vi "PH_ImageCoG_Plotter.panel.vi"(0 "object ref":refnum<vi>, 5 "error in (no error)":errorcluster) -> (19 "error out":errorcluster)   [LabVIEW 2014, in "PH_ImageCoG_Plotter.lvlib"]
doc: "The voltage measured by a device on high potential is represented by a frequency given out by a Beckhoff Klemme. This VI transforms it back into a voltage which wich is written to a memory tag. This value is indicated. In case of no connection (not mounted or bad tag value) or internal problems \"99999\" apears.\n\n\"Exit\" closes the GUI while \"Delete Instance\" additionally destroys the Instance.\n\n\n\nLicense Agreement for this software:\n\nCopyright (C)\nGesellschaft für Schwerionenforschung, GSI\nPlanckstr. 1\n64291 Darmstadt\nGermany\n\nContact: D.Beck@gsi.de \n\nThis program is free software; you can redistribute it and/or modify it under the terms of the GNU General Public License as published by the Free Software Foundation; either version 2 of the license, or (at your option) any later version.\n\nThis program is distributed in the hope that it will be useful, but WITHOUT ANYW ARRANTY; without even the implied warranty of MERCHANTABILITY or FITNESS FOR A PARTICULAR PURPOSE. See the GNU General License for more details (http://www.gnu.org).\n\nGesellschaft für Schwerionenforschung, GSI\nPlanckstr. 1, 64291 Darmstadt, Germany\nFor all questions and ideas contact: M.Richter@gsi.de, H.Brand@gsi.de or D.Beck@gsi.de.\nLast update: 18-DEC-2002"
uses:
  PH_ImageCoG_Plotter.lvlib
  PH_ImageCalibrator/PH_ImageCalibrator.Calibration Data.ctl
  PH_Basics/PH_Img_BaseClass/PH_Img_BaseClass.Palette.ctl
  PH_Basics/PH_Img_BaseClass/PH_Img_BaseClass.GUI Refs.ctl
  CS_Core/CSObj/CSObj.lvlib
  CS_Core/CSSystem/CSSystemLib/CSSystemLib.lvlib
  PH_Basics/PH_Common/PH_Common.lvlib
  PH_Basics/PH_Img_BaseClass/PH_Img_BaseClass.lvlib
  PH_Basics/PH_Class/PH_Class.lvlib
  PH_ImageCalibrator/PH_ImageCalibrator.lvlib
panel:
  in  "Export Data":bool
  out "BI subtracted":u32(colorbox)=16860 caption="BI subtr."
  out "Calibration status":u32(colorbox)=16860 caption="Calibration"
  out "Timeout":u32(colorbox)=16860
  in  "Tab Control":T1(tab)
  in  "Refresh Cam Search":bool caption="Refresh"
  in  "Available Cams":u16(ring)
  in  "Timeout Set":i32 caption="ms"
  out "Delta - X":dbl caption="Pix"
  out "Delta - Y":dbl caption="Pix"
  in  "Center":bool
  in  "exp - Y":i32 caption="Pix"
  in  "exp - X":i32 caption="Pix"
  in  "Type":bool caption="NF       FF"
  out "CoG - Y":dbl caption="Pix"
  out "CoG - X":dbl caption="Pix"
  in  "calc Beam Analysis":bool caption="On"
  out "CoG Y":cluster{dbl[], dbl[]}[](graph)
  out "CoG X":cluster{dbl[], dbl[]}[](graph)
  out "Delta Y":cluster{dbl[], dbl[]}[](graph)
  out "Delta X":cluster{dbl[], dbl[]}[](graph)
  in  "Palette":T2 items=["Grey", "Binary", "Gradient", "Rainbow", "Temperature"]
  out "GUI Image":T3(plugin-control)
  in  "read calibration data":bool
  out "Calibration data":T4
  in  "Exit":bool
  in  "Delete":bool
  # "PCS"
  # "3.40"
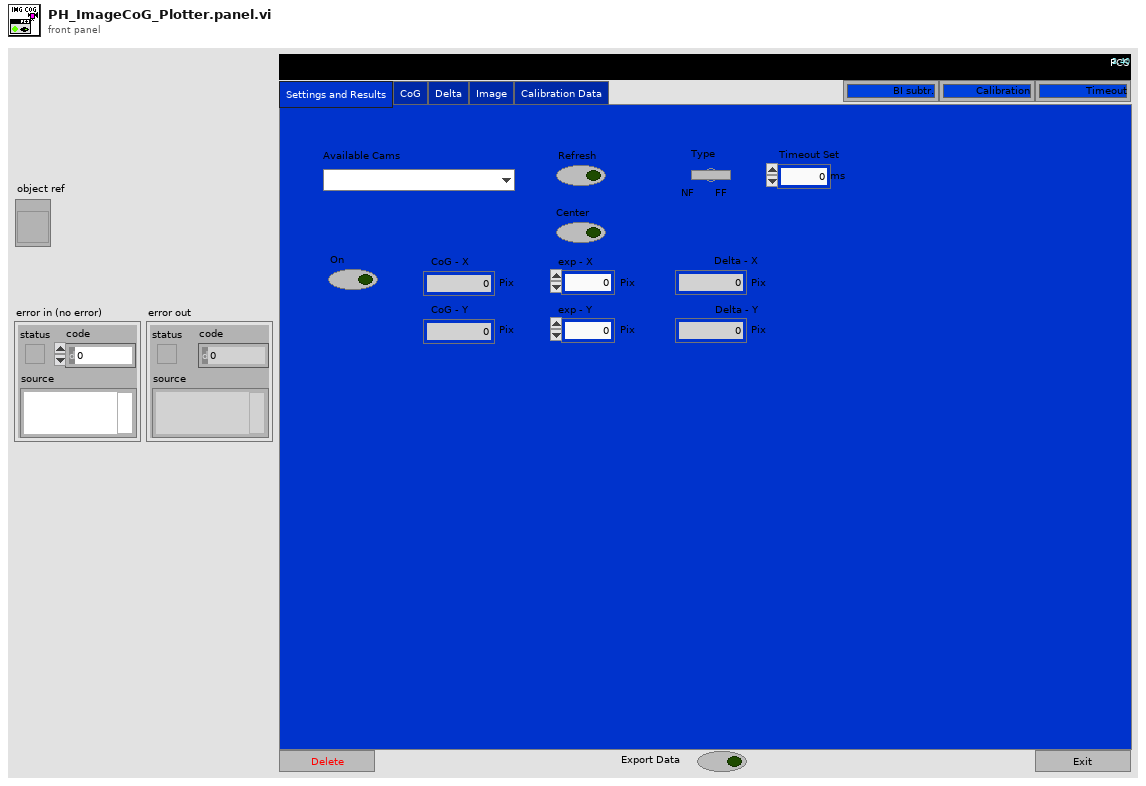
[diagram p1: front panel]
types:
  T1 = enum32{"Settings and Results", "CoG", "Delta", "Image", "Calibration Data"}
  T2 = typedef "PH_Img_BaseClass.lvlib/PH_Img_BaseClass.Palette.ctl" = i32
  T3 = typedef "IMAQ Image.ctl" = refnum<image>
  T4 = typedef "PH_ImageCalibrator.lvlib/PH_ImageCalibrator.Calibration Data.ctl" = cluster{"Date":string, "Time":string, "Cam Settings":cluster{"Cam ID":string, "Gain":dbl, "Brightness":dbl, "Shutter":dbl, "Cam Error":bool, "Mode":i32}, "Background Image":cluster{"Image":dbl[][], "Image Error":bool}, "Linear Calibration":cluster{"Calibration Factor":dbl, "not mm or mrad":bool}, "Energy Calibration":cluster{"Calibration Factor":dbl, "no mJ":bool}}
  T5 = typedef "PH_Img_BaseClass.lvlib/PH_Img_BaseClass.GUI Refs.ctl" = cluster{"Timeout":refnum<vi>, "Image":refnum<vi>, "Palette":refnum<vi>, "Timeout Set":refnum<vi>}
  T6 = typedef "PH_ImageCoG_Plotter.lvlib/PH_ImageCoG_Plotter.i attribute.ctl" = cluster{"GUI Refs":cluster{"Delete":refnum<vi>, "Calibration status":refnum<vi>, "BI subtracted":refnum<vi>, "calc Beam Anal":refnum<vi>, "CoG - x":refnum<vi>, "CoG - y":refnum<vi>, "Type":refnum<vi>, "Center":refnum<vi>, "exp - X":refnum<vi>, "exp - Y":refnum<vi>, "Delta - X":refnum<vi>, "Delta - Y":refnum<vi>, "Available Cams":refnum<vi>, "CoG X":refnum<vi>, "CoG Y":refnum<vi>, "Delta X":refnum<vi>, "Delta Y":refnum<vi>, "Export Data":refnum<vi>, "Calibration data":refnum<vi>}, "Calibration":cluster{"Status":T7, "Calibration data":T4, "Calibration Data File":path}, "Beam Analysis":cluster{"on":bool, "exp - X":i32, "exp - Y":i32, "Type":bool, "Data":cluster{"current time":timestamp, "CoG-x":dbl, "CoG-y":dbl, "Delta-x":dbl, "Delta-y":dbl}[], "Datasets strored":i32, "Dataarray Size":i32}, "Cam instances":string[], "DIM Service Events":T8[], "Images":cluster{"Background":T3, "OP":T3, "GUI":T3}}
  T7 = typedef "PH_StatusHandler.lvlib/PH_StatusHandler.Status.ctl" = i16
  T8 = typedef "BaseProcess.lvlib/BaseProcess.event definition.ctl" = cluster{"CAEEvtDef":T9, "Data Descriptor":T10}
  T9 = typedef "CAEObj.lvlib/CAEObj.event definition.ctl" = cluster{"URL":string, "enable":bool, "ignoreResID":bool}
  T10 = typedef "BaseProcess.lvlib/BaseProcess.descriptor string definition.ctl" = string
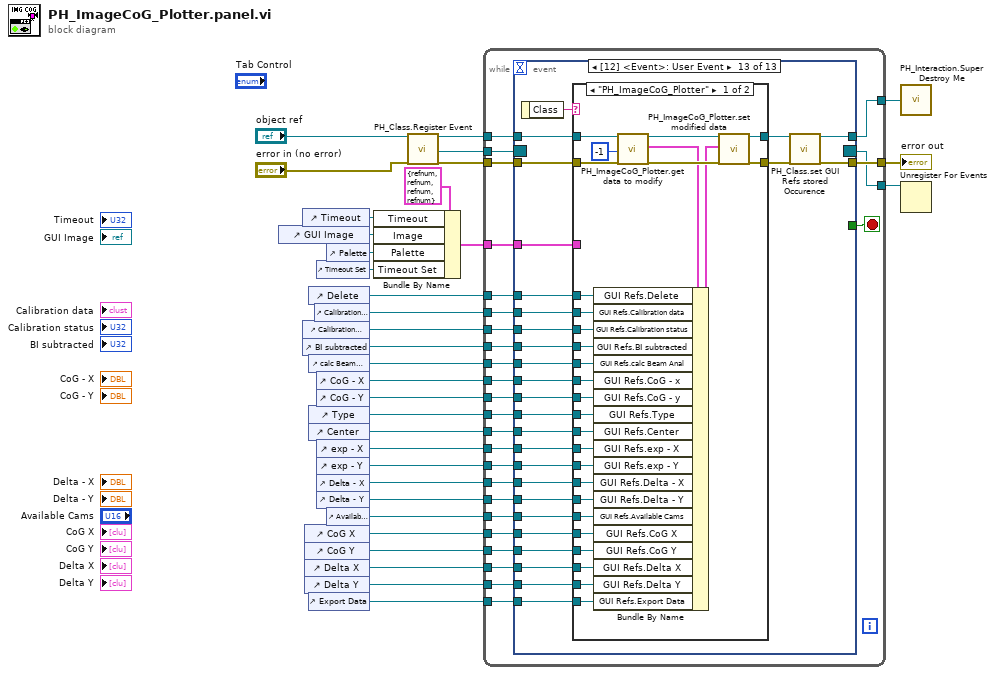
[diagram p0: block diagram]
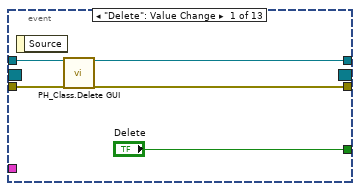
[diagram p2: hidden frame]
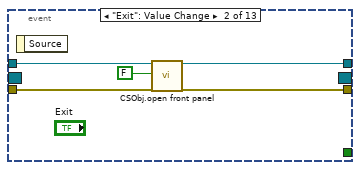
[diagram p3: hidden frame]
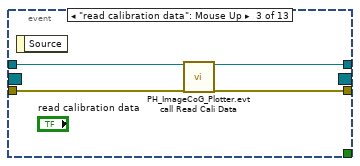
[diagram p4: hidden frame]
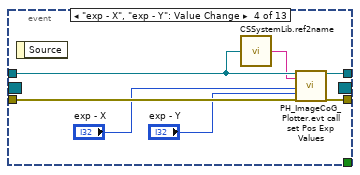
[diagram p5: hidden frame]
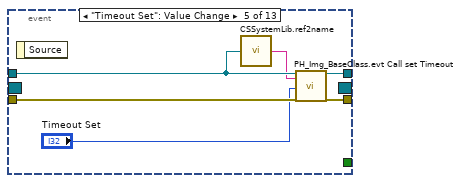
[diagram p6: hidden frame]
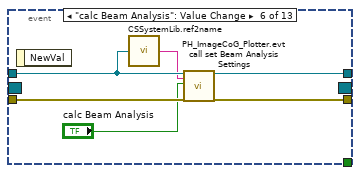
[diagram p7: hidden frame]
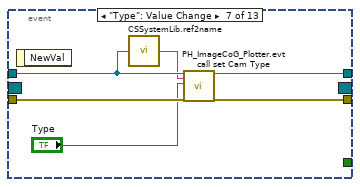
[diagram p8: hidden frame]
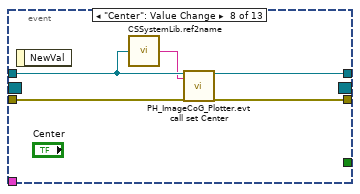
[diagram p9: hidden frame]
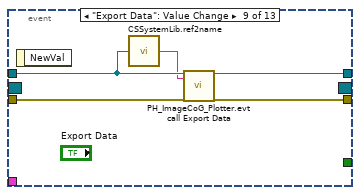
[diagram p10: hidden frame]
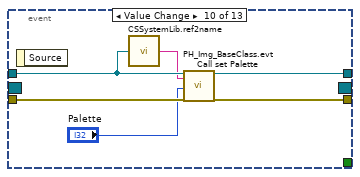
[diagram p11: hidden frame]
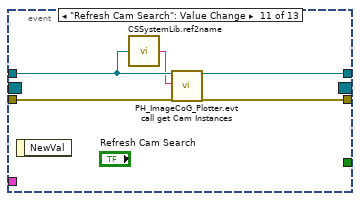
[diagram p12: hidden frame]
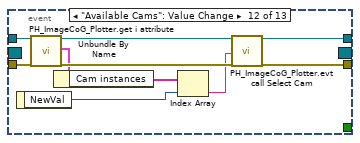
[diagram p13: hidden frame]
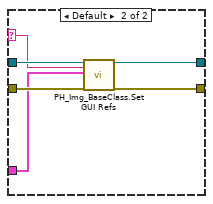
[diagram p14: hidden frame]
diagram:
  n1 = control-ref of="GUI Image"() -> (w29:refnum<vi>)
  n2 = control-ref of="Timeout"() -> (w30:refnum<vi>)
  n3 = control-ref of="Calibration status"() -> (w17:refnum<vi>)
  n4 = control-ref of="BI subtracted"() -> (w16:refnum<vi>)
  n5 = control-ref of="CoG X"() -> (w5:refnum<vi>)
  n6 = control-ref of="CoG Y"() -> (w4:refnum<vi>)
  n7 = control-ref of="Delta X"() -> (w3:refnum<vi>)
  n8 = control-ref of="Delta Y"() -> (w2:refnum<vi>)
  n9 = control-ref of="Delete"() -> (w21:refnum<vi>)
  n10 = control-ref of="calc Beam Analysis"() -> (w15:refnum<vi>)
  n11 = control-ref of="Type"() -> (w12:refnum<vi>)
  n12 = control-ref of="Center"() -> (w11:refnum<vi>)
  n13 = control-ref of="Export Data"() -> (w1:refnum<vi>)
  n14 = control-ref of="Calibration data"() -> (w18:refnum<vi>)
  n15 = control-ref of="Timeout Set"() -> (w27:refnum<vi>)
  n16 = control-ref of="CoG - X"() -> (w14:refnum<vi>)
  n17 = control-ref of="CoG - Y"() -> (w13:refnum<vi>)
  n18 = control-ref of="exp - X"() -> (w10:refnum<vi>)
  n19 = control-ref of="exp - Y"() -> (w9:refnum<vi>)
  n20 = control-ref of="Delta - X"() -> (w8:refnum<vi>)
  n21 = control-ref of="Delta - Y"() -> (w7:refnum<vi>)
  n22 = control-ref of="Palette"() -> (w28:refnum<vi>)
  n23 = control-ref of="Available Cams"() -> (w6:refnum<vi>)
  n24 = Bundle By Name(cluster=T5 {"Timeout"=refnum, "Image"=refnum, "Palette"=refnum, "Timeout Set"=refnum} ("GUI Refs"), "Timeout"=w30, "Image"=w29, "Palette"=w28, "Timeout Set"=w27) -> (w22:T5)
  n25 = call "PH_Class.Register Event.vi"("i ref in"="object ref", "error in (no error)"="error in (no error)") -> ("i ref out"=w26:refnum<vi>, "Event Registration Refnum"=w24:refnum<event-registration>, "error out"=w25:errorcluster)  [unwired: 15 in]
  n26 = while {
    tunnel: w26 -> [w57]
    tunnel: [w56] -> w33
    tunnel: w25 -> [w59]
    tunnel: [w58] -> w32
    tunnel: w24 -> [w55]
    tunnel: [w54] -> w23
    tunnel: w22 -> [w53]
    tunnel: w21 -> [w52]
    tunnel: w18 -> [w51]
    tunnel: w17 -> [w50]
    tunnel: w16 -> [w49]
    tunnel: w15 -> [w48]
    tunnel: w14 -> [w47]
    tunnel: w13 -> [w46]
    tunnel: w12 -> [w45]
    tunnel: w11 -> [w44]
    tunnel: w10 -> [w43]
    tunnel: w9 -> [w42]
    tunnel: w8 -> [w41]
    tunnel: w7 -> [w40]
    tunnel: w6 -> [w39]
    tunnel: w5 -> [w38]
    tunnel: w4 -> [w37]
    tunnel: w3 -> [w36]
    tunnel: w2 -> [w35]
    tunnel: w1 -> [w34]
    stop <- w60 stop-if-true
    n27 = event shown="[12] <Event>: User Event" {
      selector: w55 -> [_ _ _ _ _ _ _ _ _ _ _ _ _]
      dyn-events: [_ _ _ _ _ _ _ _ _ _ _ _ _] -> w54
      timeout: _ -> [_ _ _ _ _ _ _ _ _ _ _ _ _]
      tunnel: ["Delete" _ _ _ _ _ _ _ _ _ _ _ _] -> w60
      tunnel: w57 -> [w64 w69 w74 w78 w84 w90 w96 w101 w106 w112 w118 w128 w157]
      tunnel: w59 -> [w63 w68 w73 w81 w87 w93 w99 w104 w109 w115 w117 w126 w156]
      tunnel: [w61 w67 w71 w79 w85 w91 w97 w102 w107 w113 w120 w129 w149] -> w58
      tunnel: [w62 w66 w72 w80 w86 w92 w98 w103 w108 w114 w119 w130 w150] -> w56
      tunnel: w53 -> [_ _ _ _ _ _ _ _ _ _ _ _ w155]
      tunnel: w52 -> [_ _ _ _ _ _ _ _ _ _ _ _ w153]
      tunnel: w51 -> [_ _ _ _ _ _ _ _ _ _ _ _ w148]
      tunnel: w50 -> [_ _ _ _ _ _ _ _ _ _ _ _ w147]
      tunnel: w49 -> [_ _ _ _ _ _ _ _ _ _ _ _ w146]
      tunnel: w48 -> [_ _ _ _ _ _ _ _ _ _ _ _ w145]
      tunnel: w47 -> [_ _ _ _ _ _ _ _ _ _ _ _ w144]
      tunnel: w46 -> [_ _ _ _ _ _ _ _ _ _ _ _ w143]
      tunnel: w45 -> [_ _ _ _ _ _ _ _ _ _ _ _ w142]
      tunnel: w44 -> [_ _ _ _ _ _ _ _ _ _ _ _ w141]
      tunnel: w43 -> [_ _ _ _ _ _ _ _ _ _ _ _ w140]
      tunnel: w42 -> [_ _ _ _ _ _ _ _ _ _ _ _ w139]
      tunnel: w41 -> [_ _ _ _ _ _ _ _ _ _ _ _ w138]
      tunnel: w40 -> [_ _ _ _ _ _ _ _ _ _ _ _ w137]
      tunnel: w39 -> [_ _ _ _ _ _ _ _ _ _ _ _ w136]
      tunnel: w38 -> [_ _ _ _ _ _ _ _ _ _ _ _ w135]
      tunnel: w37 -> [_ _ _ _ _ _ _ _ _ _ _ _ w134]
      tunnel: w36 -> [_ _ _ _ _ _ _ _ _ _ _ _ w133]
      tunnel: w35 -> [_ _ _ _ _ _ _ _ _ _ _ _ w132]
      tunnel: w34 -> [_ _ _ _ _ _ _ _ _ _ _ _ w131]
      event "Delete": Value Change {
        n28 = event-data() -> ()  [unwired: 1 in, 1 out]
        n29 = call "PH_Class.Delete GUI.vi"("VI in"=w64, "error in (no error)"=w63) -> ("VI out"=w62:refnum<vi>, "error out"=w61:errorcluster)  [unwired: 16 in]
      }
      event "Exit": Value Change {
        n30 = event-data() -> ()  [unwired: 1 in, 1 out]
        n31 = call "CSObj.open front panel.vi"("i ref in"=w69, "frontPanelOpen"=FALSE ("front panel open"), "error in (no error)"=w68) -> ("i ref out"=w66:refnum<vi>, "error out"=w67:errorcluster)  [unwired: 15 in]
      }
      event "read calibration data": Mouse Up {
        n32 = event-data() -> ()  [unwired: 1 in, 1 out]
        n33 = call "PH_ImageCoG_Plotter.evt call Read Cali Data.vi"("i ref in"=w74, "error in"=w73) -> ("i ref out"=w72:refnum<vi>, "error out"=w71:errorcluster)  [unwired: 16 in]
      }
      event "exp - X", "exp - Y": Value Change {
        n34 = event-data() -> ()  [unwired: 1 in, 1 out]
        n35 = call "CSSystemLib.ref2name.vi"("obj refnum"=w78) -> ("name"=w77:string)
        n36 = call "PH_ImageCoG_Plotter.evt call set Pos Exp Values.vi"("i ref in"=w78, "Instance"=w77, "expected value  x [Pix]"="exp - X", "expected value y [Pix]"="exp - Y", "error in (no error)"=w81) -> ("i ref out"=w80:refnum<vi>, "error out"=w79:errorcluster)  [unwired: 13 in]
      }
      event "Timeout Set": Value Change {
        n37 = event-data() -> ()  [unwired: 1 in, 1 out]
        n38 = call "CSSystemLib.ref2name.vi"("obj refnum"=w84) -> ("name"=w83:string)
        n39 = call "PH_Img_BaseClass.evt Call set Timeout.vi"("i ref in"=w84, "Instance"=w83, "Timeout [ms]"="Timeout Set", "error in (no error)"=w87) -> ("i ref out"=w86:refnum<vi>, "error out"=w85:errorcluster)  [unwired: 14 in]
      }
      event "calc Beam Analysis": Value Change {
        n40 = event-data() -> ()  [unwired: 1 in, 1 out]
        n41 = call "CSSystemLib.ref2name.vi"("obj refnum"=w90) -> ("name"=w89:string)
        n42 = call "PH_ImageCoG_Plotter.evt call set Beam Analysis Settings.vi"("i ref in"=w90, "Instance"=w89, "Calculate"="calc Beam Analysis", "error in (no error)"=w93) -> ("i ref out"=w92:refnum<vi>, "error out"=w91:errorcluster)  [unwired: 14 in]
      }
      event "Type": Value Change {
        n43 = event-data() -> ()  [unwired: 1 in, 1 out]
        n44 = call "CSSystemLib.ref2name.vi"("obj refnum"=w96) -> ("name"=w95:string)
        n45 = call "PH_ImageCoG_Plotter.evt call set Cam Type.vi"("i ref in"=w96, "Instance"=w95, "Cam Type"="Type", "error in (no error)"=w99) -> ("i ref out"=w98:refnum<vi>, "error out"=w97:errorcluster)  [unwired: 14 in]
      }
      event "Center": Value Change {
        n46 = event-data() -> ()  [unwired: 1 in, 1 out]
        n47 = call "CSSystemLib.ref2name.vi"("obj refnum"=w101) -> ("name"=w100:string)
        n48 = call "PH_ImageCoG_Plotter.evt call set Center.vi"("i ref in"=w101, "Instance"=w100, "error in (no error)"=w104) -> ("i ref out"=w103:refnum<vi>, "error out"=w102:errorcluster)  [unwired: 15 in]
      }
      event "Export Data": Value Change {
        n49 = event-data() -> ()  [unwired: 1 in, 1 out]
        n50 = call "CSSystemLib.ref2name.vi"("obj refnum"=w106) -> ("name"=w105:string)
        n51 = call "PH_ImageCoG_Plotter.evt call Export Data.vi"("i ref in"=w106, "Instance"=w105, "error in (no error)"=w109) -> ("i ref out"=w108:refnum<vi>, "error out"=w107:errorcluster)  [unwired: 15 in]
      }
      event Value Change {
        n52 = event-data() -> ()  [unwired: 1 in, 1 out]
        n53 = call "CSSystemLib.ref2name.vi"("obj refnum"=w112) -> ("name"=w111:string)
        n54 = call "PH_Img_BaseClass.evt Call set Palette.vi"("i ref in"=w112, "Instance"=w111, "Palette"="Palette", "error in (no error)"=w115) -> ("i ref out"=w114:refnum<vi>, "error out"=w113:errorcluster)  [unwired: 14 in]
      }
      event "Refresh Cam Search": Value Change {
        n55 = event-data() -> ()  [unwired: 1 in, 1 out]
        n56 = call "CSSystemLib.ref2name.vi"("obj refnum"=w118) -> ("name"=w116:string)
        n57 = call "PH_ImageCoG_Plotter.evt call get Cam Instances.vi"("i ref in"=w118, "Object"=w116, "error in (no error)"=w117) -> ("i ref out"=w119:refnum<vi>, "error out"=w120:errorcluster)  [unwired: 15 in]
      }
      event "Available Cams": Value Change {
        n58 = event-data() -> ("NewVal"=w122:u16)  [unwired: 1 in]
        n59 = call "PH_ImageCoG_Plotter.get i attribute.vi"("i ref in"=w128, "error in (no error)"=w126) -> ("i ref out"=w127:refnum<vi>, "i attribute"=w124:T6, "error out"=w125:errorcluster)  [unwired: 15 in]
        n60 = Unbundle By Name(w124) -> ("Cam instances"=w123:string[])
        n61 = Index Array(array=w123, index=w122) -> (element=w121:string)
        n62 = call "PH_ImageCoG_Plotter.evt call Select Cam.vi"("i ref in"=w127, "Cam"=w121, "error in"=w125) -> ("i ref out"=w130:refnum<vi>, "error out"=w129:errorcluster)  [unwired: 15 in]
      }
      event User Event {
        n63 = event-data() -> ("Class"=w154:string)  [unwired: 1 in]
        n64 = case shown="\"PH_ImageCoG_Plotter\"" w154 {
          selector: w154 -> [_ w186]
          tunnel: w157 -> [w182 w191]
          tunnel: w156 -> [w181 w190]
          tunnel: [w179 w189] -> w151
          tunnel: [w180 w188] -> w152
          tunnel: w155 -> [_ w187]
          tunnel: w153 -> [w178 _]
          tunnel: w148 -> [w175 _]
          tunnel: w147 -> [w174 _]
          tunnel: w146 -> [w173 _]
          tunnel: w145 -> [w172 _]
          tunnel: w144 -> [w171 _]
          tunnel: w143 -> [w170 _]
          tunnel: w142 -> [w169 _]
          tunnel: w141 -> [w168 _]
          tunnel: w140 -> [w167 _]
          tunnel: w139 -> [w166 _]
          tunnel: w138 -> [w165 _]
          tunnel: w137 -> [w164 _]
          tunnel: w136 -> [w163 _]
          tunnel: w135 -> [w162 _]
          tunnel: w134 -> [w161 _]
          tunnel: w133 -> [w160 _]
          tunnel: w132 -> [w159 _]
          tunnel: w131 -> [w158 _]
          frame "PH_ImageCoG_Plotter" {
            n65 = call "PH_ImageCoG_Plotter.get data to modify.vi"("i ref in"=w182, "ms timeout (10000)"=-1, "error in (no error)"=w181) -> ("i ref out"=w183:refnum<vi>, "i attribute"=w177:T6, "error out"=w184:errorcluster)  [unwired: 13 in, 1 out]
            n66 = Bundle By Name(cluster=w177, "GUI Refs.Delete"=w178, "GUI Refs.Calibration data"=w175, "GUI Refs.Calibration status"=w174, "GUI Refs.BI subtracted"=w173, "GUI Refs.calc Beam Anal"=w172, "GUI Refs.CoG - x"=w171, "GUI Refs.CoG - y"=w170, "GUI Refs.Type"=w169, "GUI Refs.Center"=w168, "GUI Refs.exp - X"=w167, "GUI Refs.exp - Y"=w166, "GUI Refs.Delta - X"=w165, "GUI Refs.Delta - Y"=w164, "GUI Refs.Available Cams"=w163, "GUI Refs.CoG X"=w162, "GUI Refs.CoG Y"=w161, "GUI Refs.Delta X"=w160, "GUI Refs.Delta Y"=w159, "GUI Refs.Export Data"=w158) -> (w176:T6)
            n67 = call "PH_ImageCoG_Plotter.set modified data.vi"("i ref in"=w183, "i attribute"=w176, "error in (no error)"=w184) -> ("i ref out"=w180:refnum<vi>, "error out"=w179:errorcluster)  [unwired: 15 in]
          }
          frame Default {
            n68 = call "PH_Img_BaseClass.Set GUI Refs.vi"("i ref in"=w191, "Class"=w186, "GUI Refs"=w187, "error in (no error)"=w190) -> ("i ref out"=w188:refnum<vi>, "error out"=w189:errorcluster)  [unwired: 14 in]
          }
        }
        n69 = call "PH_Class.set GUI Refs stored Occurence.vi"("i ref in"=w152, "error in (no error)"=w151) -> ("i ref out"=w150:refnum<vi>, "error out"=w149:errorcluster)  [unwired: 16 in]
      }
    }
  }
  "error out" <- w32
  n70 = call "PH_Interaction.Super Destroy Me.vi"("i ref out"=w33) -> ()
  n71 = Unregister For Events(event registration refnum=w23) -> ()  [unwired: 1 in, 1 out]
